vi "Initialize.vi"(8 "error in (no error)":errorcluster, 11 "DemoCamera in":refnum<class "DemoCamera.lvclass">) -> (0 "error out":errorcluster, 3 "DemoCamera out":refnum<class "DemoCamera.lvclass">)   [LabVIEW 2020, in "DemoCamera.lvlib" / "DemoCamera.lvclass"]
uses:
  DemoCamera.lvclass
  Hardware Abstraction Layer/Component/Camera/Camera/Camera.lvclass
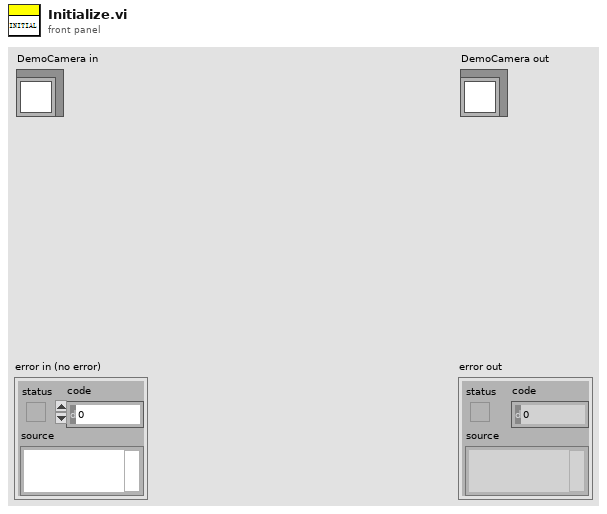
[diagram p1: front panel]
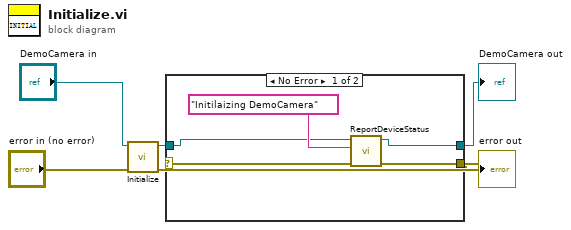
[diagram p0: block diagram]
diagram:
  n1 = call-parent "Initialize.vi"("error in (no error)"="error in (no error)", "Camera in"="DemoCamera in") -> ("error out"=w4:errorcluster, "Camera out"=w2:refnum<class "DemoCamera.lvclass">)  [unwired: 8 in]
  n2 = case shown="No Error" w4 {
    selector: w4 -> [w9 w13]
    tunnel: [w11 w13] -> w3
    tunnel: w2 -> [w8 w12]
    tunnel: [w7 w12] -> w1
    frame No Error {
      n3 = call-dynamic "ReportDeviceStatus.vi"("error in (no error)"=w9, "Status"="Initilaizing DemoCamera", "Device in"=w8) -> ("error out"=w11:errorcluster, "Device out"=w7:refnum<class "DemoCamera.lvclass">)  [unwired: 7 in]
    }
    frame Error {
    }
  }
  "error out" <- w3
  "DemoCamera out" <- w1
